vi "example_GMessage.vi"() -> ()   [LabVIEW 2020]
uses:
  <vilib>/Galil/resources/gclib32/gclib32.lvlib
panel:
  in  "?":bool
  out "Messages":string
  in  "Program":string="#test\nMG \"Sample Number:\",TIME\nWT 10\nJP#test\n"
  out "Error Out":errorcluster
  in  "IP Address":string="192.168.1.77 -s MG"
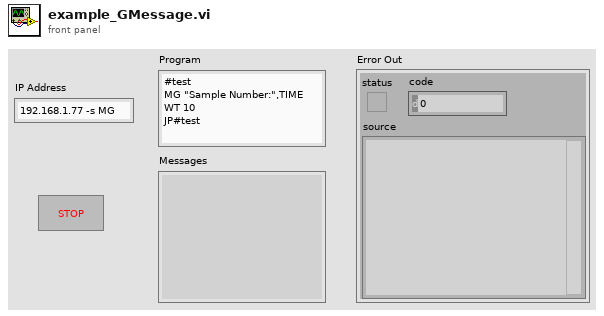
[diagram p1: front panel]
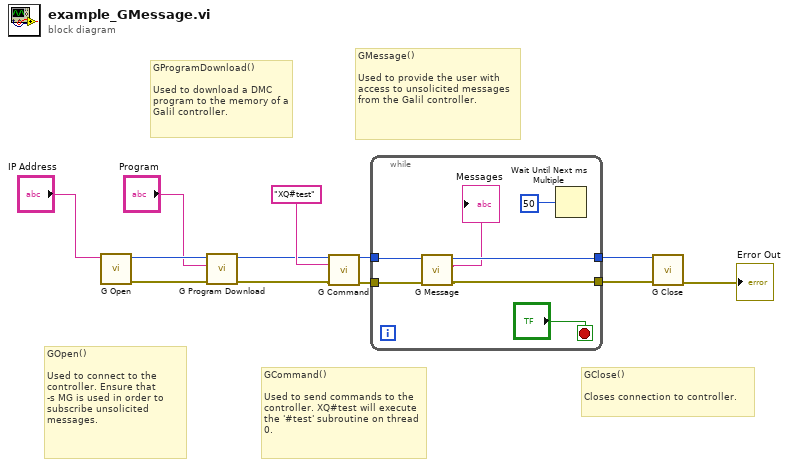
[diagram p0: block diagram]
diagram:
  # "GClose()\n\nCloses connection to controller."
  # "GMessage()\n\nUsed to provide the user with access to unsolicited messages from the Galil controller."
  # "GCommand()\n\nUsed to send commands to the controller. XQ#test will execute the '#test' subroutine on thread 0."
  # "GProgramDownload()\n\nUsed to download a DMC  program to the memory of a Galil controller."
  # "GOpen()\n\nUsed to connect to the controller. Ensure that \n-s MG is used in order to subscribe unsolicited messages."
  n1 = call <vilib>:"G Open.vi"("address"="IP Address") -> ("error out"=w3:errorcluster, "g out"=w5:u32)  [unwired: 8 in]
  n2 = call <vilib>:"G Program Download.vi"("error in (no error)"=w3, "program"="Program", "g"=w5) -> ("error out"=w2:errorcluster, "g out"=w1:u32)  [unwired: 7 in]
  n3 = call <vilib>:"G Command.vi"("g"=w1, "command"="XQ#test", "error in (no error)"=w2) -> ("g out"=w9:u32, "error out"=w7:errorcluster)  [unwired: 10 in, 1 out]
  n4 = while {
    tunnel: w9 -> [w17]
    tunnel: [w15] -> w11
    tunnel: w7 -> [w16]
    tunnel: [w13] -> w10
    stop <- "?" stop-if-true
    n5 = call <vilib>:"G Message.vi"("error in (no error)"=w16, "g"=w17) -> ("error out"=w13:errorcluster, "buffer out"=→"Messages":string, "g out"=w15:u32)  [unwired: 7 in]
    n6 = Wait Until Next ms Multiple(millisecond multiple=u32 50) -> ()  [unwired: 1 out]
  }
  n7 = call <vilib>:"G Close.vi"("error in (no error)"=w10, "g"=w11) -> ("error out"=→"Error Out":errorcluster)  [unwired: 9 in]
